vi "scan_array_2D_super.vi"(5 "v1_config":T1={"hardware"=enum."none", "options"="", "repeats"=1, "loops"=1, "VISA"="", "override_VISA"=FALSE} {"loops" min=1; "repeats" min=1}, 7 "v0_config":T1={"hardware"=enum."none", "options"="", "repeats"=1, "loops"=1, "VISA"="", "override_VISA"=FALSE} {"loops" min=1; "repeats" min=1}, 8 "error in":errorcluster, 9 "var mode":enum16{"permutations", "aligned"}(ring), 10 "v1_values":dbl[](array[numeric])=[1.0, 2.0, 3.0, 4.0, 5.0, 6.0, 7.0, 8.0, 9.0, 10.0] format="%#_6p", 11 "v0_values":dbl[](array[numeric])=[1.0, 2.0, 3.0, 4.0, 5.0, 6.0, 7.0, 8.0, 9.0, 10.0] format="%#_6p") -> (0 "error in (no error)":errorcluster={"status"=TRUE, "code"=999, "source"="Failed to align var arrays\nof different length"}, 2 "scan_values":dbl[][](array[numeric]))   [LabVIEW 2017, in "tools.lvlib"]
uses:
  tools.lvlib
  var_config.ctl
  ctrl/var_list.ctl
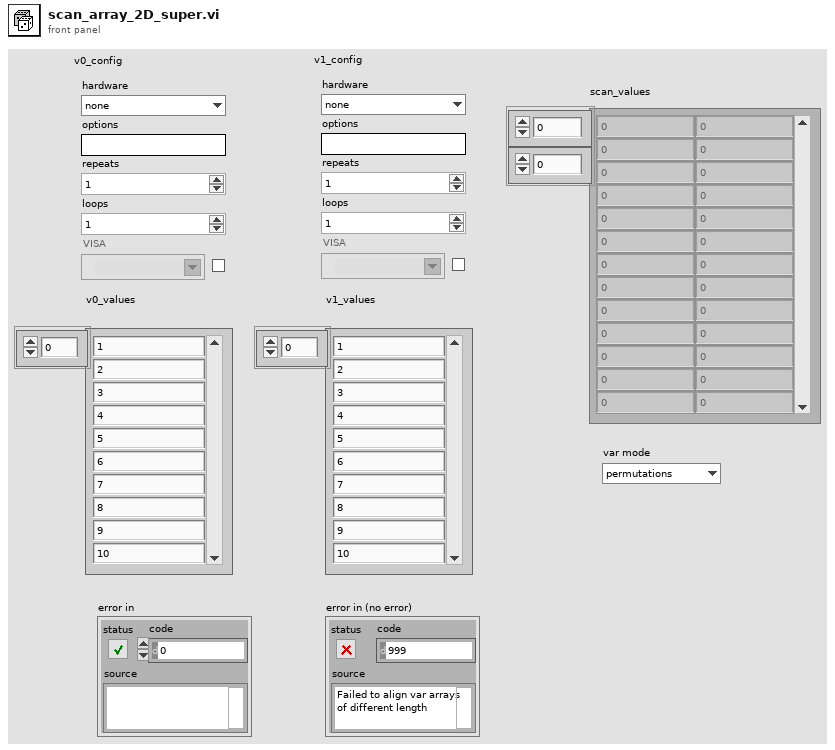
[diagram p1: front panel]
types:
  T1 = typedef "tools.lvlib/var_config.ctl" = cluster{"hardware":T2, "options":string, "repeats":i32, "loops":i32, "VISA":refnum<visa-resource-name>, "override_VISA":bool}
  T2 = typedef "var_list.ctl" = enum16{"none", "AO voltage (V)", "delay (s)", "generic", "microwaves (GHz)", "radiant (nm)", "radiant thg (nm)", "sirah (nm)", "sirah_shg (nm)", "tenma voltage (V)", "wait (s)", "wf_freq (Hz)", "wf_amp (V)", "wf_amp_multi (V)", "wf_offset (V)", "wf_low_level (V)", "wf_high_level (V)", "wf_period (s)", "wf_pulse_width (s)", "wf_sample_rate (Sa/s)", "wf_multi_amp", "wf_multi_freq", "wf_arb_4chan", "WS7 setpoint (nm)"}
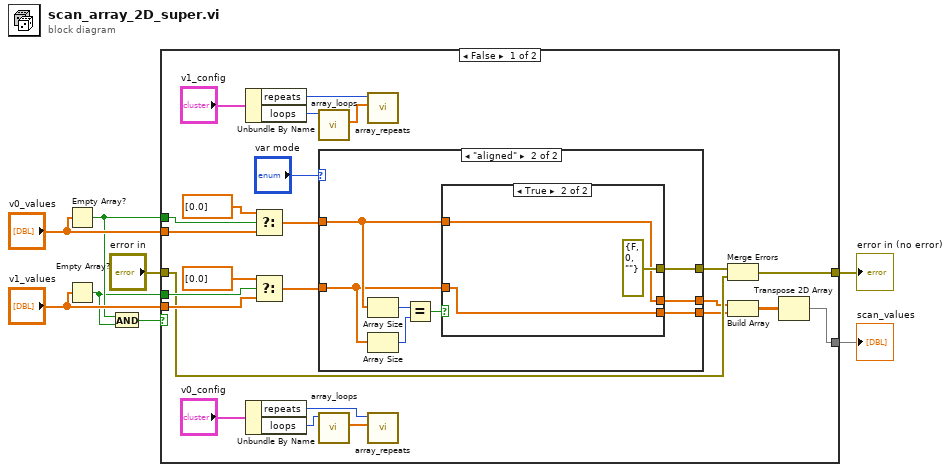
[diagram p0: block diagram]
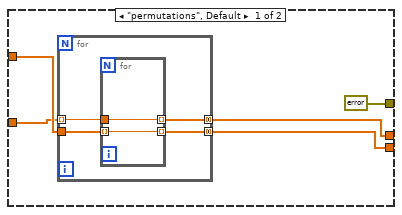
[diagram p2: hidden frame]
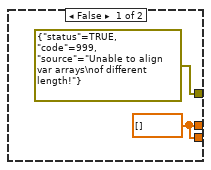
[diagram p3: hidden frame]
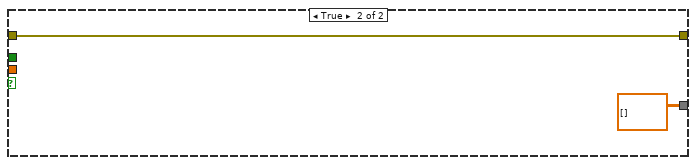
[diagram p4: hidden frame]
diagram:
  n1 = Empty Array?(array="v0_values") -> (empty?=w5:bool)
  n2 = Empty Array?(array="v1_values") -> (empty?=w4:bool)
  n3 = And(x=w5, y=w4) -> (x .and. y?=w1:bool)
  n4 = case shown="False" w1 {
    tunnel: [w25 w58] -> w8
    tunnel: "v1_values" -> [w22 _]
    tunnel: "v0_values" -> [w21 _]
    tunnel: w5 -> [w19 _]
    tunnel: w4 -> [w18 _]
    tunnel: [w10 dbl[][] []] -> w3
    tunnel: "error in" -> [w17 w58]
    frame False {
      n5 = Unbundle By Name("v1_config") -> ("repeats"=w31:i32, "loops"=w27:i32)
      n6 = Unbundle By Name("v0_config") -> ("repeats"=w29:i32, "loops"=w28:i32)
      n7 = Select(t=dbl[] [0.0], s=w19, f=w21) -> (s? t:f=w9:dbl[])
      n8 = Select(t=dbl[] [0.0], s=w18, f=w22) -> (s? t:f=w14:dbl[])
      n9 = call "array_loops.vi"("loops"=w27) -> ("values_OUT"=w16:dbl[])  [unwired: 10 in]
      n10 = case shown="\"aligned\"" "var mode" {
        tunnel: [w34 w45] -> w11
        tunnel: w9 -> [w37 w48]
        tunnel: w14 -> [w36 w47]
        tunnel: [errorcluster {"status"=FALSE, "code"=0, "source"=""} ("error in (no error)") w46] -> w24
        tunnel: [w33 w44] -> w12
        frame "permutations", Default {
          n11 = for {
            tunnel: w37 -> [w41]
            tunnel: w36 -> [w40] mode=indexing
            tunnel: [w39] -> w34 mode=concatenating
            tunnel: [w38] -> w33 mode=concatenating
            n12 = for {
              tunnel: w41 -> [w43] mode=indexing
              tunnel: w40 -> [w42]
              tunnel: [w43] -> w39 mode=indexing
              tunnel: [w42] -> w38 mode=indexing
            }
          }
        }
        frame "aligned" {
          n13 = Array Size(array=w48) -> (size(s)=w51:i32)
          n14 = Array Size(array=w47) -> (size(s)=w50:i32)
          n15 = Equal?(x=w51, y=w50) -> (x = y?=w49:bool)
          n16 = case shown="True" w49 {
            tunnel: [w52 w55] -> w45
            tunnel: w48 -> [_ w54]
            tunnel: w47 -> [_ w55]
            tunnel: [errorcluster {"status"=TRUE, "code"=999, "source"="Unable to align var arrays\nof different length!"} ("error in (no error)") errorcluster {"status"=FALSE, "code"=0, "source"=""} ("error in (no error)")] -> w46
            tunnel: [w52 w54] -> w44
            frame False {
              w52 = dbl[] []
            }
            frame True {
            }
          }
        }
      }
      n17 = call "array_loops.vi"("loops"=w28) -> ("values_OUT"=w15:dbl[])  [unwired: 10 in]
      n18 = call "array_repeats.vi"("values_IN"=w16, "repeats"=w31) -> ()  [unwired: 9 in, 1 out]
      n19 = call "array_repeats.vi"("values_IN"=w15, "repeats"=w29) -> ()  [unwired: 9 in, 1 out]
      n20 = Merge Errors(w24, w17) -> (w25:errorcluster)
      n21 = Build Array(w12, w11) -> (w13:dbl[][])
      n22 = Transpose 2D Array(2D array=w13) -> (transposed array=w10:dbl[][])
    }
    frame True {
    }
  }
  "error in (no error)" <- w8
  "scan_values" <- w3
